vi "AlazarStackChannels5Pass.vi"(4 "lines per plane":i32, 6 "AlazarCluster":T5, 7 "Digitizer Settings":T1 {"Trigger Settings"."Trig Slope" items=["Positive", "Negative"]; "Trigger Settings"."Level (mV)" format="%.2f"; "Trigger Settings"."Trig Coupling" items=["DC 1 MOhm", "AC 1 MOhm", "DC 50 Ohm", "AC 50 Ohm"]; "Trigger Settings"."Trig Source" items=["Chan 1", "External"]; "Rel Dig Delay" format="%.2f"; "DigTimeOut" format="%.2f"; "Avg Num" min=1; "Offset delay (us)" format="%.2f"; "Additional dig delay (us)" format="%.2f"; "Digitizer delay (us)" format="%.2f"}, 8 "error in":errorcluster, 9 "Channels":i32, 10 "Extra Shift":u16) -> (0 "error out":errorcluster, 1 "Voltage Scale":dbl, 2 "Return Code":u32, 3 "ChStackDataOut":i16[][][](array[numeric]))   [LabVIEW 2022 SP3]
uses:
  -DigitizerRoutines/DigitizerSettings.ctl
  -DigitizerRoutines/Digitizer.ctl
  -DigitizerRoutines/DigConfig.ctl
  -DigitizerRoutines/DigitizerID.ctl
  C:/Windows/System32/ADQAPI_dotNet_helper.dll
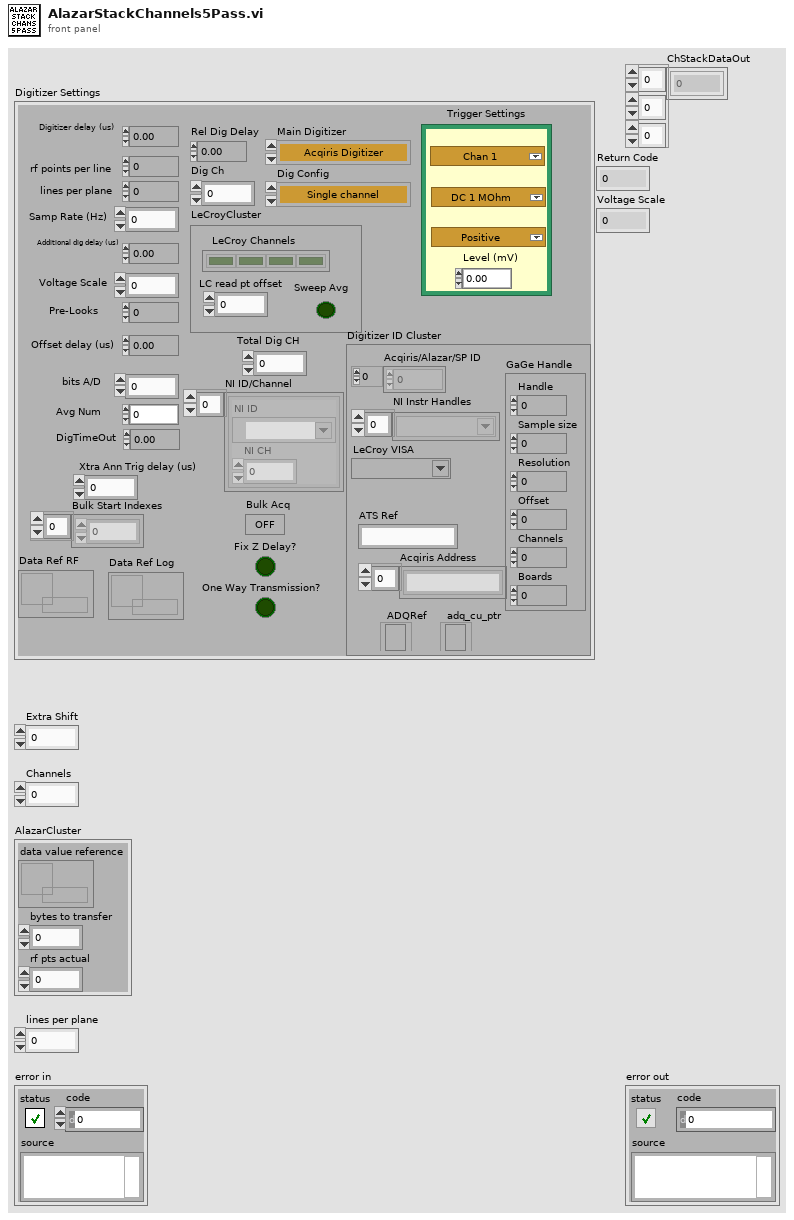
[diagram p1: front panel]
types:
  T1 = typedef "DigitizerSettings.ctl" = cluster{"Digitizer delay (us) ":dbl, "rf points per line":i32, "lines per plane":i32, "Samp Rate (Hz)":dbl, "Additional dig delay (us)":dbl, "Voltage Scale":dbl, "Pre-Looks":i32, "Offset delay (us)":dbl, "bits A/D":i8, "Avg Num":i32, "DigTimeOut":sgl, "Rel Dig Delay":sgl, "Dig Ch":i32, "LeCroyCluster":cluster{"LeCroy Channels":bool[], "LC read pt offset":dbl, "Sweep Avg":bool}, "Main Digitizer":T2, "Dig Config":T3, "Digitizer ID Cluster":T4, "Trigger Settings":cluster{"Trig Source":u16, "Trig Coupling":u16, "Trig Slope":u16, "Level (mV)":dbl}, "Bulk Acq":bool, "Bulk Start Indexes":i32[], "Data Ref RF":refnum<data-value>, "NI ID/Channel":cluster{"NI ID":refnum<k15>, "NI CH":i32}[], "Total Dig CH":i32, "Xtra Ann Trig delay (us)":dbl, "Fix Z Delay?":bool, "One Way Transmission?":bool, "Data Ref Log":refnum<data-value>}
  T2 = typedef "Digitizer.ctl" = enum16{"Acqiris Digitizer", "NI Digitizer", "LeCroy", "GaGe", "AlazarTech", "No Digitizer", "Teledyne"}
  T3 = typedef "DigConfig.ctl" = enum16{"Single channel", "2 Chans w/ 2 Acqiris", "2 Chans w/ 1 Acqiris", "5-CH Pulser New", "5-CH pulser w/ ann array", "5-pass style ann array", "Empty"}
  T4 = typedef "DigitizerID.ctl" = cluster{"Acqiris/Alazar/SP ID":u32[], "NI Instr Handles":refnum<k15>[], "LeCroy VISA":refnum<visa-resource-name>, "GaGe Handle":cluster{"Handle":u32, "Sample size":u32, "Resolution":i32, "Offset":i32, "Channels":u32, "Boards":u32}, "ATS Ref":string, "Acqiris Address":string[], "ADQRef":refnum<k24>, "adq_cu_ptr":refnum<k24>}
  T5 = cluster{"data value reference":refnum<data-value>, "bytes to transfer":u32, "rf pts actual":u32}
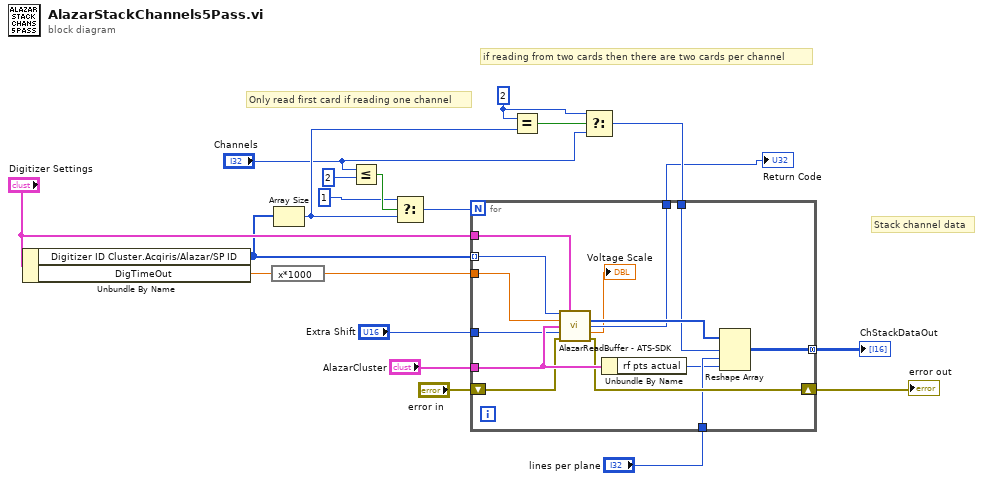
[diagram p0: block diagram]
diagram:
  w5 = 2 ("y")
  # "Stack channel data"
  # "if reading from two cards then there are two cards per channel"
  # "Only read first card if reading one channel"
  n1 = Unbundle By Name("Digitizer Settings") -> ("Digitizer ID Cluster.Acqiris/Alazar/SP ID"=w11:u32[], "DigTimeOut"=w12:sgl)
  n2 = expression code="x*1000"(w12) -> (w16:sgl)
  n3 = Array Size(array=w11) -> (size(s)=w7:i32)
  n4 = Less Or Equal?(x="Channels", y=2) -> (x <= y?=w10:bool)
  n5 = Select(t=1 ("y"), s=w10, f=w7) -> (s? t:f=w8:i32)
  n6 = Equal?(x=w5, y=w7) -> (x = y?=w6:bool)
  n7 = Select(t=w5, s=w6, f="Channels") -> (s? t:f=w3:i32)
  n8 = for {
    N: w8 -> [_]
    tunnel: "AlazarCluster" -> [w34]
    tunnel: "Extra Shift" -> [w31]
    tunnel: w16 -> [w29]
    tunnel: w3 -> [w28]
    tunnel: "lines per plane" -> [w27]
    tunnel: [w25] -> w14 mode=concatenating
    tunnel: "Digitizer Settings" -> [w24]
    tunnel: w11 -> [w23] mode=indexing
    shift-right: [w33] -> w19
    shift-left: "error in" -> [w32]
    tunnel: [w22] -> w2
    n9 = call "AlazarReadBuffer - ATS-SDK.vi"("Handle"=w23, "Digitizer Settings"=w24, "time out (ms)"=w29, "AlazarCluster"=w34, "Extra Shift"=w31, "error in (no error)"=w32) -> ("Data Array"=w30:i16[], "Return Code"=w22:u32, "Voltage Scale"=→"Voltage Scale":dbl, "error out"=w33:errorcluster)  [unwired: 5 in, 1 out]
    n10 = Unbundle By Name(w34) -> ("rf pts actual"=w26:u32)
    n11 = Reshape Array(w30, w28, w27, w26) -> (w25:i16[][][])
  }
  "error out" <- w19
  "ChStackDataOut" <- w14
  "Return Code" <- w2
